vi "DidInit.vi"(8 "ErrorArray In":errorcluster[](array[cluster]), 10 "Init?":bool, 11 "NISTBus In":refnum<class "NISTBus.lvclass">) -> (0 "ErrorArray Out":errorcluster[](array[cluster]), 3 "NISTBus Out":refnum<class "NISTBus.lvclass">)   [LabVIEW 2014, in "Bus.lvlib"]
uses:
  Bus.lvlib
  NISTBus.lvclass
  Typedefs/clDidInit.ctl
  Typedefs/clUserEventType.ctl
  <userlib>/NIST/NISTErrorLib/NISTErrorLib.lvlib
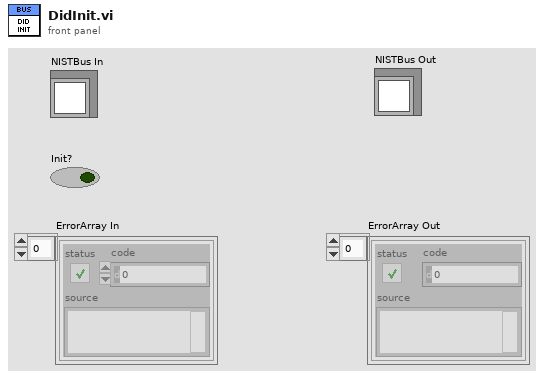
[diagram p1: front panel]
types:
  T1 = typedef "Bus.lvlib/clUserEventType.ctl" = cluster{"BusNumber":i8, "Data":variant}
  T2 = typedef "Bus.lvlib/clDidInit.ctl" = cluster{"NISTBus":refnum<vi>, "Init?":bool}
  T3 = typedef "Bus.lvlib/clBroadcastEvents.ctl" = cluster{"DidInit":refnum<user-event>, "DidStop":refnum<user-event>}
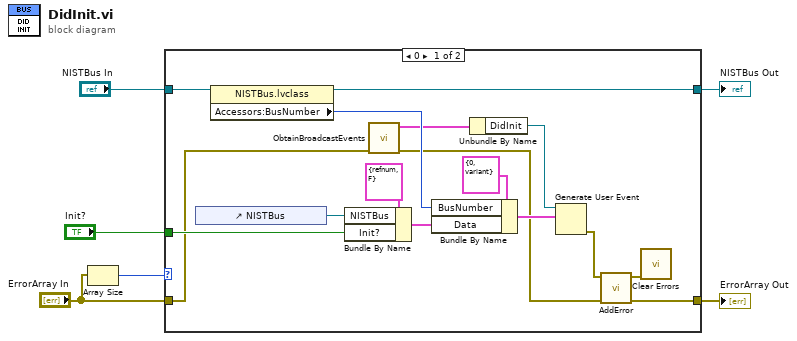
[diagram p0: block diagram]
diagram:
  n1 = Array Size(array="ErrorArray In") -> (size(s)=w4:i32)
  n2 = case shown="0" w4 {
    tunnel: "NISTBus In" -> [w22 w24]
    tunnel: [w21 w24] -> w5
    tunnel: "ErrorArray In" -> [w14 w23]
    tunnel: [w11 w23] -> w2
    tunnel: "Init?" -> [w18 _]
    frame 0 {
      n3 = control-ref of="NISTBus"() -> (w19:refnum<vi>)
      n4 = property class="NISTBus.lvclass"(reference=w22) -> (reference out=w21:refnum<class "NISTBus.lvclass">, "Accessors:BusNumber"=w15:u8)  [unwired: 1 in, 1 out]
      n5 = Bundle By Name(cluster=T2 {"NISTBus"=refnum, "Init?"=FALSE} ("clNISTBusDidInit"), "NISTBus"=w19, "Init?"=w18) -> (w16:T2)
      n6 = call "ObtainBroadcastEvents.vi"("ErrorArray In"=w14) -> ("ErrorArray Out"=w7:errorcluster[], "NISTBusBroadcast"=w9:T3)  [unwired: 9 in]
      n7 = Bundle By Name(cluster=T1 {"BusNumber"=0, "Data"=variant} ("clEventType"), "BusNumber"=w15, "Data"=w16) -> (w10:T1)
      n8 = Unbundle By Name(w9) -> ("DidInit"=w8:refnum<user-event>)
      n9 = Generate User Event(user event=w8, event data cluster=w10) -> (error out=w13:errorcluster)  [unwired: 2 in, 1 out]
      n10 = call <userlib>:"AddError.vi"("ErrorArray"=w7, "error in (no error)"=w13) -> ("ErrorArray"=w11:errorcluster[], "error out"=w12:errorcluster)  [unwired: 8 in]
      n11 = call <vilib>:"Clear Errors.vi"("error in (no error)"=w12) -> ()  [unwired: 5 in, 2 out]
    }
    frame 1, Default {
    }
  }
  "NISTBus Out" <- w5
  "ErrorArray Out" <- w2
